vi "Open & Set TWM.vi"(8 "error in":errorcluster, 11 "QPS settings":T1={"TWM pipe name"="\\\\.\\pipe\\TWM:server", "Measurement properties"={"Measurement ID"=enum."1", "Description"="3 phase, 3 ADC, 1 PJVS", "Switching matrix M"=[], "Signal frequency  (Hz)"=50.0, "Signal amplitudes (V)"=[], "PRs"=1, "PRe"=10, "MRs"=0, "MRe"=0, "Set PJVS frequency (Hz)"=50.0, "PJVS reference voltages (1 period, V)"=[], "Requiested PJVS steps"=10, "Sampling f (Hz)"=7000.0}, "PJVS setup"={"PJVS type"=enum."AC-supraVOLTcontrol", "Status Refnum"=refnum, "Abort Refnum"=refnum, "AC-supraVOLTcontrol"={"IP address:port (0.0.0.0:0000)"="0.0.0.0:0000", "Timeouts"={"TCP Read & Write (ms)"=7000, "Sensors readout"=5000, "PJVS setup"=10000, "Nullmeter readout"=5000, "Multiplexer setup"=3000, "57XX setup"=15000, "Generator setup"=5000, "Synthesizer setup"=3000, "Sampler readout"=10000}, "Simulation mode"=FALSE, "Debug mode"=FALSE}, "NPL bias source"={"Server name"="CZC", "Bias setup file"=path ""}}} {"Measurement properties"."PJVS reference voltages (1 period, V)" format="%.9g"}) -> (0 "error out":errorcluster, 2 "TWM handle out":i32, 3 "QPS settings out":T1={"TWM pipe name"="\\\\.\\pipe\\TWM:server", "Measurement properties"={"Measurement ID"=enum."1", "Description"="3 phase, 3 ADC, 1 PJVS", "Switching matrix M"=[], "Signal frequency  (Hz)"=50.0, "Signal amplitudes (V)"=[], "PRs"=1, "PRe"=10, "MRs"=0, "MRe"=0, "Set PJVS frequency (Hz)"=50.0, "PJVS reference voltages (1 period, V)"=[], "Requiested PJVS steps"=10, "Sampling f (Hz)"=7000.0}, "PJVS setup"={"PJVS type"=enum."AC-supraVOLTcontrol", "Status Refnum"=refnum, "Abort Refnum"=refnum, "AC-supraVOLTcontrol"={"IP address:port (0.0.0.0:0000)"="0.0.0.0:0000", "Timeouts"={"TCP Read & Write (ms)"=7000, "Sensors readout"=5000, "PJVS setup"=10000, "Nullmeter readout"=5000, "Multiplexer setup"=3000, "57XX setup"=15000, "Generator setup"=5000, "Synthesizer setup"=3000, "Sampler readout"=10000}, "Simulation mode"=FALSE, "Debug mode"=FALSE}, "NPL bias source"={"Server name"="CZC", "Bias setup file"=path ""}}} {"Measurement properties"."PJVS reference voltages (1 period, V)" format="%.9g"})   [LabVIEW 2020]
uses:
  external libraries/TWM client.lvlibp
  external libraries/TWM client.lvlibp/server/TWM client/TWM Client Processing Setup.ctl
  external libraries/TWM client.lvlibp/server/TWM client/TWM Client Meas Setup.ctl
  Type definitions/Measurement ID.ctl
  Type definitions/Measuement properties.ctl
  General PJVS driver/Type definitions/PJVS Type.ctl
  PJVS drivers/acsvcontrol-driver/build/ACSVcontrol-driver_0.2.0.0.llb/Timeouts.ctl
  PJVS drivers/acsvcontrol-driver/build/ACSVcontrol-driver_0.2.0.0.llb/ACSVcontrol-driver.lvlib
  General PJVS driver/Type definitions/PJVS Setup.ctl
  General PJVS driver/QPSsettings.ctl
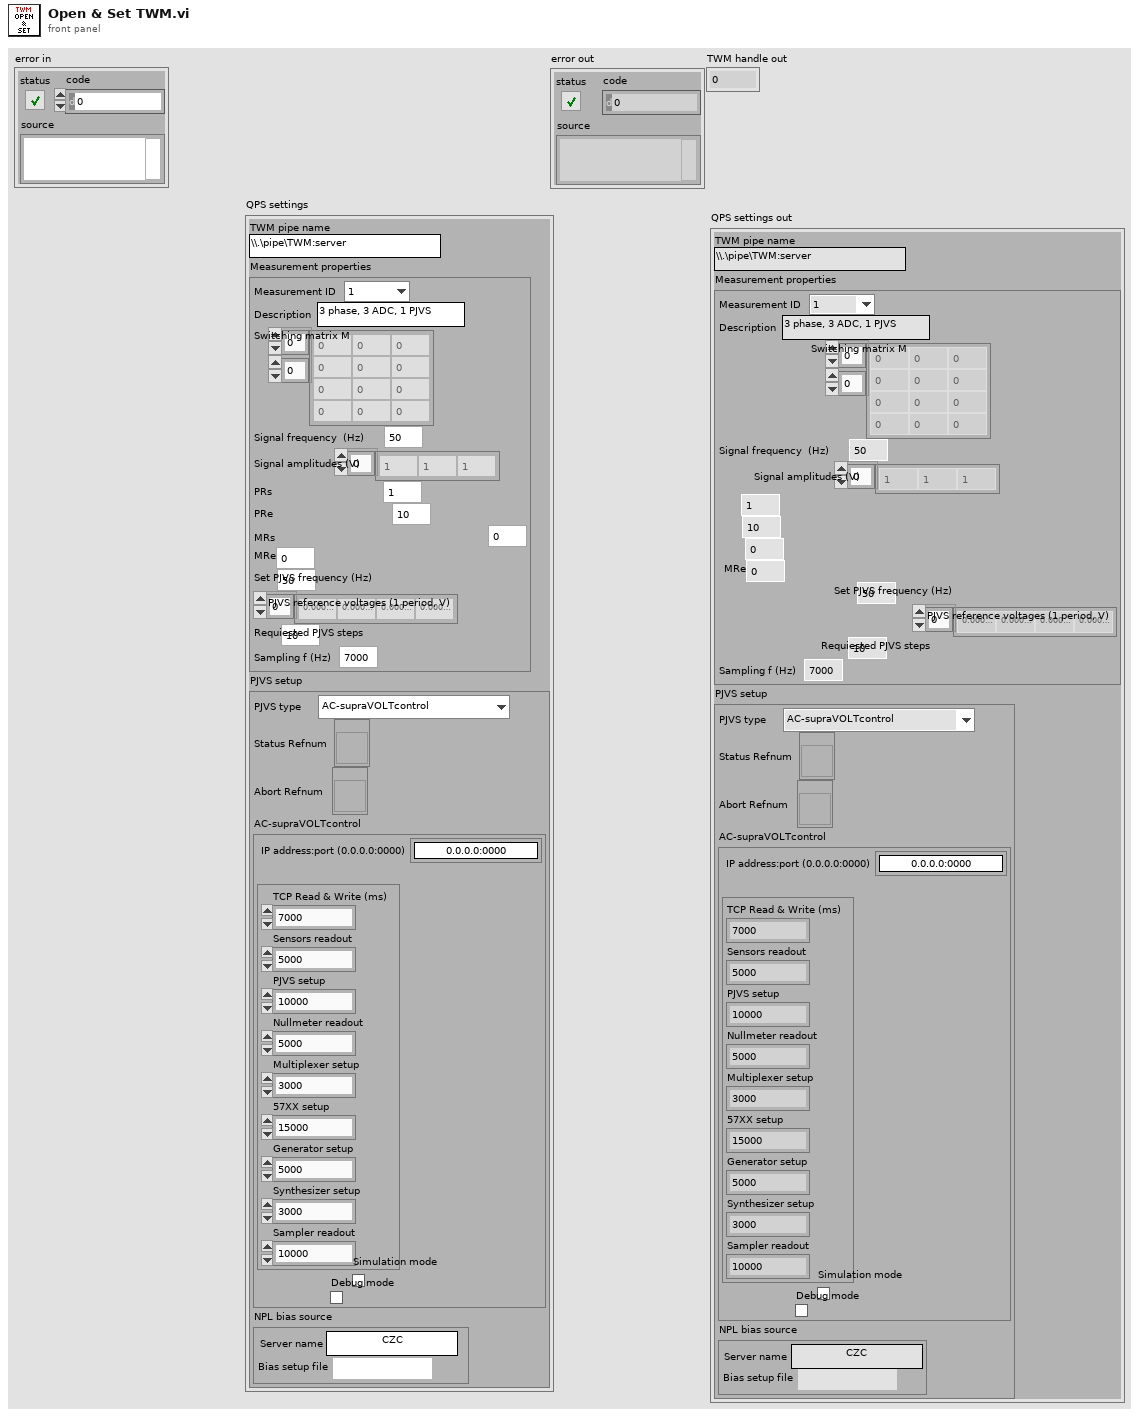
[diagram p1: front panel]
types:
  T1 = typedef "QPSsettings.ctl" = cluster{"TWM pipe name":string, "Measurement properties":T2, "PJVS setup":T4}
  T2 = typedef "Measuement properties.ctl" = cluster{"Measurement ID":T3, "Description":string, "Switching matrix M":i32[][], "Signal frequency  (Hz)":dbl, "Signal amplitudes (V)":dbl[], "PRs":i32, "PRe":i32, "MRs":i32, "MRe":i32, "Set PJVS frequency (Hz)":dbl, "PJVS reference voltages (1 period, V)":dbl[], "Requiested PJVS steps":i32, "Sampling f (Hz)":dbl}
  T3 = typedef "Measurement ID.ctl" = enum16{"M", "1", "2", "3"}
  T4 = typedef "PJVS Setup.ctl" = cluster{"PJVS type":T5, "Status Refnum":refnum<vi>, "Abort Refnum":refnum<vi>, "AC-supraVOLTcontrol":cluster{"IP address:port (0.0.0.0:0000)":string, "Timeouts":T6, "Simulation mode":bool, "Debug mode":bool}, "NPL bias source":cluster{"Server name":string, "Bias setup file":path}}
  T5 = typedef "PJVS Type.ctl" = enum16{"AC-supraVOLTcontrol", "NPL bias source"}
  T6 = typedef "ACSVcontrol-driver.lvlib/Timeouts.ctl" = cluster{"TCP Read & Write (ms)":i32, "Sensors readout":i32, "PJVS setup":i32, "Nullmeter readout":i32, "Multiplexer setup":i32, "57XX setup":i32, "Generator setup":i32, "Synthesizer setup":i32, "Sampler readout":i32}
  T7 = typedef "TWM client.lvlibp/TWM Client Meas Setup.ctl" = cluster{"smpl count":i32, "smpl rate [Hz]":dbl, "average":i32, "aperture [s]":dbl, "valid?":bool, "meas fld":path, "sub-records":i32, "ranges [Vpk]":dbl[], "smpl rate - fr [Hz]":dbl, "smpl rate - div":dbl, "smpl rate - mul":dbl}
  T8 = typedef "TWM client.lvlibp/TWM Client Processing Setup.ctl" = cluster{"calculate":i32, "all cycles at once":bool, "alg. ID":string, "unc mode":string, "mc cycles":i32, "timeout [s]":dbl, "loc [-]":dbl, "valid?":bool, "qwtb params":cluster{"name":string, "data":string[]}[]}
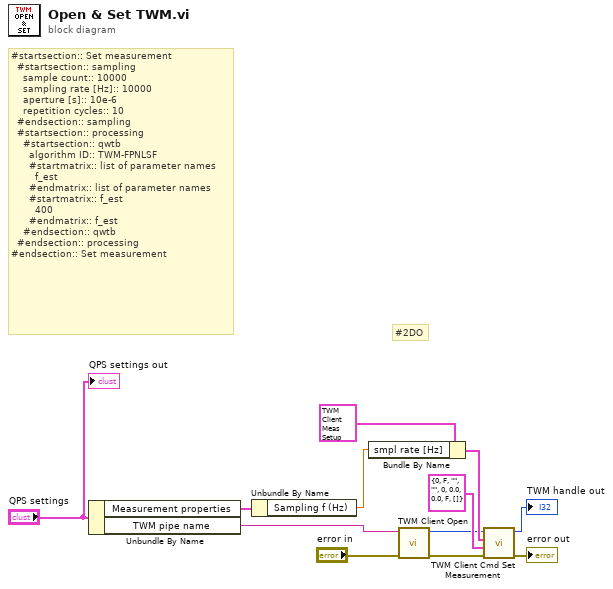
[diagram p0: block diagram]
diagram:
  # "#2DO"
  # "#startsection:: Set measurement\n  #startsection:: sampling\n    sample count:: 10000\n    sampling rate [Hz]:: 10000\n    aperture [s]:: 10e-6\n    repetition cycles:: 10\n  #endsection:: sampling\n  #startsection:: processing\n    #startsection:: qwtb\n      algorithm ID:: TWM-FPNLSF\n      #startmatrix:: list of parameter names\n        f_est\n      #endmatrix:: list of parameter names\n      #startmatrix:: f_est\n        400\n      #endmatrix:: f_est\n    #endsection:: qwtb\n  #endsection:: processing\n#endsection:: Set measurement"
  n1 = Unbundle By Name("QPS settings") -> ("Measurement properties"=w9:T2, "TWM pipe name"=w11:string)
  n2 = Unbundle By Name(w9) -> ("Sampling f (Hz)"=w5:dbl)
  n3 = Bundle By Name(cluster=T7 {"smpl count"=0, "smpl rate [Hz]"=0.0, "average"=0, "aperture [s]"=0.0, "valid?"=FALSE, "meas fld"=path "", "sub-records"=0, "ranges [Vpk]"=[], "smpl rate - fr [Hz]"=0.0, "smpl rate - div"=0.0, "smpl rate - mul"=0.0} ("meas"), "smpl rate [Hz]"=w5) -> (w4:T7)
  n4 = call "TWM Client Open.vi"("error in"="error in", "pipe name"=w11) -> ("error out"=w8:errorcluster, "handle out"=w3:i32)  [unwired: 8 in]
  n5 = call "TWM Client Cmd Set Measurement.vi"("error in"=w8, "processing"=T8 {"calculate"=0, "all cycles at once"=FALSE, "alg. ID"="", "unc mode"="", "mc cycles"=0, "timeout [s]"=0.0, "loc [-]"=0.0, "valid?"=FALSE, "qwtb params"=[]}, "meas"=w4, "handle"=w3) -> ("error out"=→"error out":errorcluster, "handle out"=→"TWM handle out":i32)  [unwired: 6 in]
  "QPS settings out" <- "QPS settings"
